vi "Error Query.vi"(8 "error in (no error)":errorcluster, 11 "VISA resource name":refnum<visa-resource-name>) -> (0 "error out":errorcluster, 1 "Error Message":string, 2 "Error Code":i32[](array[numeric]), 3 "VISA resource name out":refnum<visa-resource-name>)   [LabVIEW 2014, in "Agilent MXA Series.lvlib"]
doc: "Queries the instrument for any errors in the instrument's error queue. It will continue to read errors until all errors have been read from the instrument. Any errors will be returned in the <B>error out</B> control.\n\n<B>Note:</B>\nThis VI is called automatically by most driver VIs so it is not usually necessary to call this in an application."
uses:
  Agilent MXA Series.lvlib
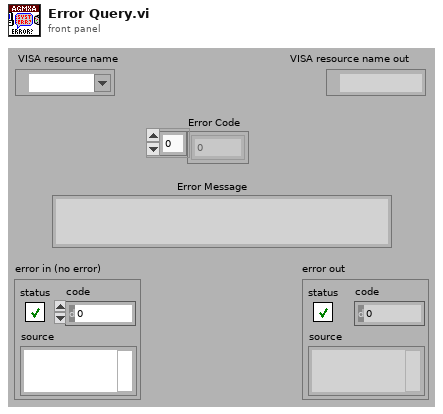
[diagram p1: front panel]
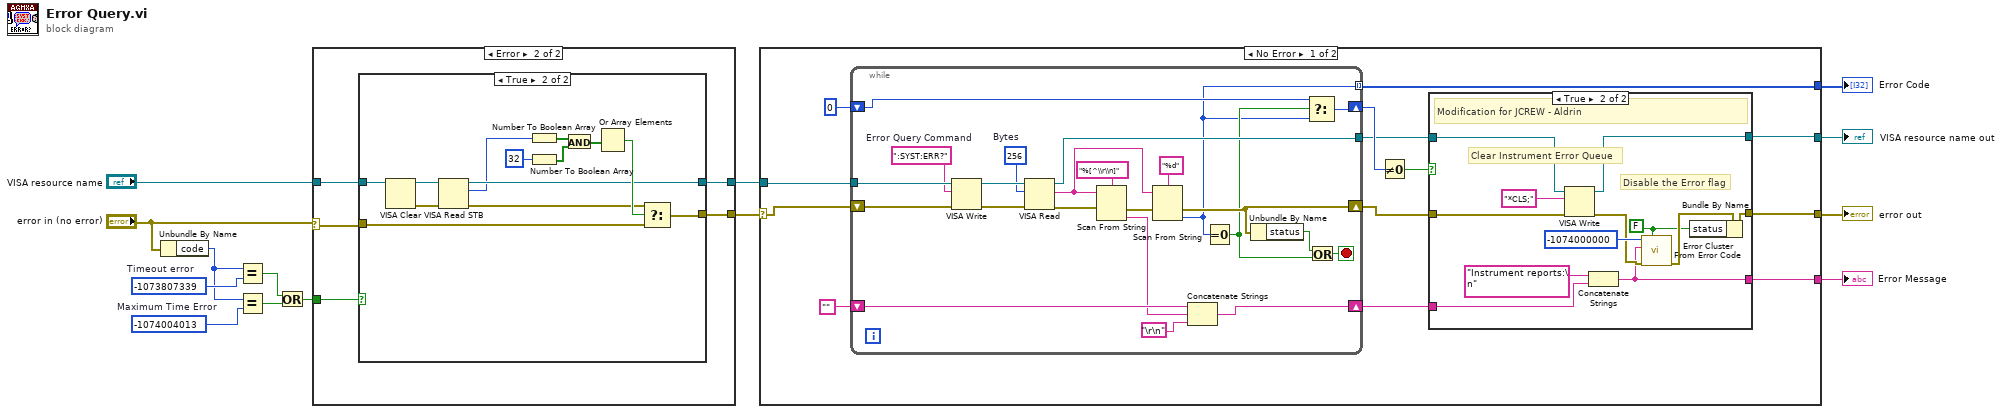
[diagram p0: block diagram]
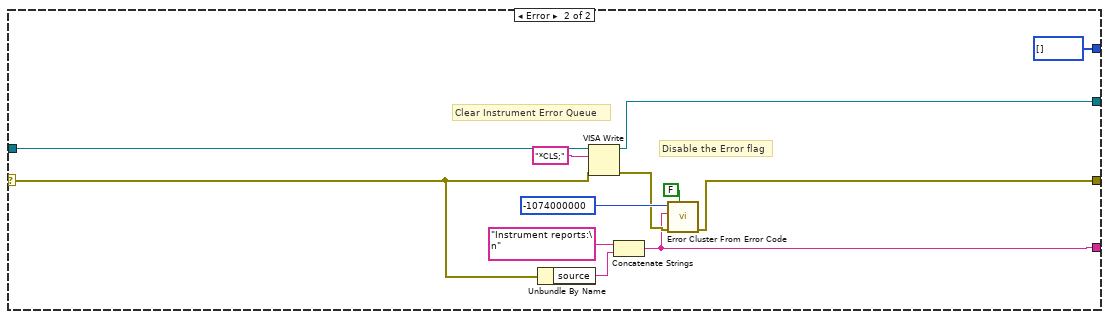
[diagram p5: hidden frame]
diagram:
  w12 = -1074004013  # Maximum Time Error
  w14 = -1073807339  # Timeout error
  n1 = Unbundle By Name("error in (no error)") -> ("code"=w13:i32)
  n2 = Equal?(x=w13, y=w14) -> (x = y?=w10:bool)
  n3 = Equal?(x=w13, y=w12) -> (x = y?=w11:bool)
  n4 = Or(x=w10, y=w11) -> (x .or. y?=w7:bool)
  n5 = case shown="Error" "error in (no error)" {
    selector: "error in (no error)" -> [w15 w19]
    tunnel: "VISA resource name" -> [w16 w21]
    tunnel: [w16 w20] -> w5
    tunnel: [w15 w18] -> w6
    tunnel: w7 -> [_ w17]
    frame No Error {
    }
    frame Error {
      n6 = case shown="True" w17 {
        tunnel: w21 -> [w23 w29]
        tunnel: [w23 w26] -> w20
        tunnel: w19 -> [w22 w32]
        tunnel: [w22 w31] -> w18
        frame False {
        }
        frame True {
          n7 = VISA Clear(VISA resource name=w29) -> (VISA resource name out=w28:refnum<visa-resource-name>, error out=w27:errorcluster)  [unwired: 1 in]
          n8 = VISA Read STB(8:w27, 11:w28) -> (0:w25:errorcluster, 2:w24:u16, 3:w26:refnum<visa-resource-name>)
          n9 = Number To Boolean Array(number=w24) -> (Boolean array=w33:bool[])
          n10 = Number To Boolean Array(number=32) -> (Boolean array=w35:bool[])
          n11 = And(x=w33, y=w35) -> (x .and. y?=w34:bool[])
          n12 = Or Array Elements(Boolean array=w34) -> (logical OR=w30:bool)
          n13 = Select(t=w25, s=w30, f=w32) -> (s? t:f=w31:errorcluster)
        }
      }
    }
  }
  n14 = case shown="No Error" w6 {
    selector: w6 -> [w44 w93]
    tunnel: [w39 w88] -> w3
    tunnel: w5 -> [w49 w89]
    tunnel: [w38 w91] -> w2
    tunnel: [w37 w90] -> w1
    tunnel: [w45 i32[] []] -> w4
    frame No Error {
      n15 = while {
        tunnel: [w87] -> w41
        tunnel: w49 -> [w86]
        shift-right: [w74] -> w43
        shift-left: "" ("Empty String Constant") -> [w77]
        shift-right: [w72] -> w46
        shift-left: 0 -> [w73]
        shift-right: [w70] -> w42
        shift-left: w44 -> [w71]
        tunnel: [w65] -> w45 mode=indexing
        stop <- w80 stop-if-true
        w84 = u32 256  # Bytes
        w82 = ":SYST:ERR?"  # Error Query Command
        n16 = VISA Write(VISA resource name=w86, write buffer=w82, error in (no error)=w71) -> (VISA resource name out=w85:refnum<visa-resource-name>, error out=w83:errorcluster)  [unwired: 1 out]
        n17 = VISA Read(VISA resource name=w85, byte count=w84, error in (no error)=w83) -> (VISA resource name out=w87:refnum<visa-resource-name>, read buffer=w78:string, error out=w69:errorcluster)  [unwired: 1 out]
        n18 = Scan From String(format string="%[^\\r\\n]", input string=w78, error in=w69) -> (error out=w68:errorcluster, output 1=w75:string)  [unwired: 1 in, 3 out]
        n19 = Scan From String(format string="%d", input string=w78, error in=w68) -> (error out=w70:errorcluster, output 1=w65:i32)  [unwired: 1 in, 3 out]
        n20 = Concatenate Strings(w77, w75, "\r\n" ("End of Line Constant")) -> (w74:string)
        n21 = Equal To 0?(x=w65) -> (x = 0?=w66:bool)
        n22 = Unbundle By Name(w70) -> ("status"=w67:bool)
        n23 = Select(t=w73, s=w66, f=w65) -> (s? t:f=w72:i32)
        n24 = Or(x=w67, y=w66) -> (x .or. y?=w80:bool)
      }
      n25 = Not Equal To 0?(x=w46) -> (x != 0?=w40:bool)
      n26 = case shown="True" w40 {
        tunnel: w43 -> [w50 w63]
        tunnel: [w52 w54] -> w38
        tunnel: w42 -> [w52 w60]
        tunnel: w41 -> [w51 w57]
        tunnel: [w51 w56] -> w39
        tunnel: [w50 w55] -> w37
        frame False {
        }
        frame True {
          w53 = FALSE ("show call chain? (False)")
          # "Disable the Error flag"
          # "Clear Instrument Error Queue"
          # "Modification for JCREW - Aldrin"
          n27 = VISA Write(VISA resource name=w57, write buffer="*CLS;", error in (no error)=w60) -> (VISA resource name out=w56:refnum<visa-resource-name>, error out=w59:errorcluster)  [unwired: 1 out]
          n28 = Concatenate Strings("Instrument reports:\n" ("Source"), w63) -> (w55:string)
          n29 = call "Error Cluster From Error Code.vi"("show call chain? (False)"=w53, "error in (no error)"=w59, "error message (\"\")"=w55, "error code (0)"=-1074000000 ("Code")) -> ("error out"=w61:errorcluster)  [unwired: 5 out]
          n30 = Bundle By Name(cluster=w61, "status"=w53) -> (w54:errorcluster)
        }
      }
    }
    frame Error {
      # "Disable the Error flag"
      # "Clear Instrument Error Queue"
      n31 = Unbundle By Name(w93) -> ("source"=w92:string)
      n32 = VISA Write(VISA resource name=w89, write buffer="*CLS;", error in (no error)=w93) -> (VISA resource name out=w88:refnum<visa-resource-name>, error out=w95:errorcluster)  [unwired: 1 out]
      n33 = Concatenate Strings("Instrument reports:\n" ("Source"), w92) -> (w90:string)
      n34 = call "Error Cluster From Error Code.vi"("show call chain? (False)"=FALSE, "error in (no error)"=w95, "error message (\"\")"=w90, "error code (0)"=-1074000000 ("Code")) -> ("error out"=w91:errorcluster)  [unwired: 5 out]
    }
  }
  "VISA resource name out" <- w3
  "error out" <- w2
  "Error Message" <- w1
  "Error Code" <- w4
